vi "Get Created Group.vi"(4 "error in (no error)":errorcluster, 6 "Group Number (1)":i32=1 min=1, 7 "VISA resource name":refnum<visa-resource-name>) -> (0 "error out":errorcluster, 2 "Axis":i32[](array[numeric]), 3 "VISA resource name out":refnum<visa-resource-name>)   [LabVIEW 2018, in "Newport ESP301.lvlib"]
doc: "this command reports the axes assigned to the group in the order of their assignment."
uses:
  Newport ESP301.lvlib
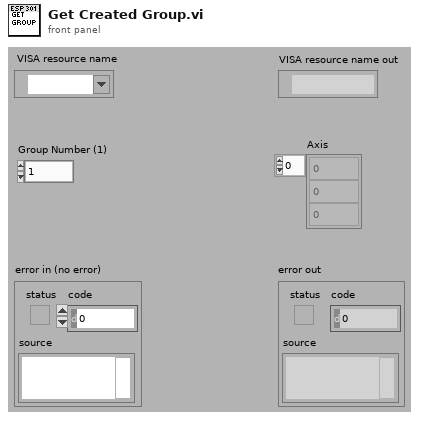
[diagram p1: front panel]
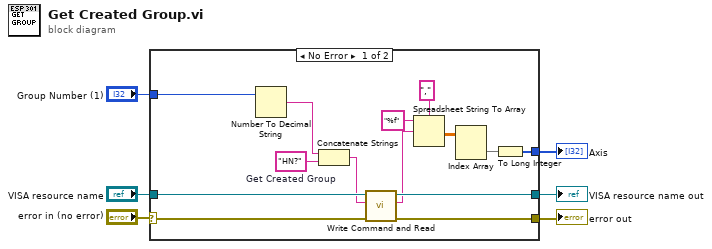
[diagram p0: block diagram]
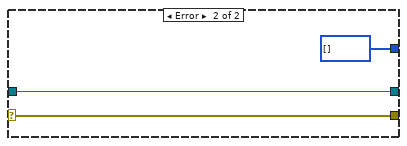
[diagram p2: hidden frame]
diagram:
  n1 = case shown="No Error" "error in (no error)" {
    selector: "error in (no error)" -> [w17 w23]
    tunnel: [w19 w23] -> w6
    tunnel: "VISA resource name" -> [w20 w22]
    tunnel: [w18 w22] -> w5
    tunnel: "Group Number (1)" -> [w13 _]
    tunnel: [w7 i32[] []] -> w1
    frame No Error {
      w16 = "HN?"  # Get Created Group
      n2 = Number To Decimal String(number=w13) -> (decimal integer string=w15:string)  [unwired: 1 in]
      n3 = Concatenate Strings(w15, w16) -> (w14:string)
      n4 = call "Write Command and Read.vi"("error in (no error)"=w17, "Command"=w14, "VISA resource name"=w20) -> ("error out"=w19:errorcluster, "Returned string"=w11:string, "VISA resource name out"=w18:refnum<visa-resource-name>)  [unwired: 4 in]
      n5 = Spreadsheet String To Array(delimiter (Tab)="," ("séparateur (Tabulation)"), format string="%f" ("chaîne de format"), spreadsheet string=w11) -> (array=w10:dbl[][])  [unwired: 1 in]
      n6 = Index Array(array=w10) -> (element=w8:dbl[])  [unwired: 2 in]
      n7 = To Long Integer(number=w8) -> (32bit integer=w7:i32[])
    }
    frame Error {
    }
  }
  "error out" <- w6
  "VISA resource name out" <- w5
  "Axis" <- w1
